vi "PhoenixLauncher.vi"() -> ()   [LabVIEW 2023]
uses:
  Vision_class/Old vision/Decode SSL and Refree Wrapper Package Folder/SSL Referee Game Status.ctl
  Vision_class/Old vision/Controls/SSL Field State.ctl
  Vision_class/Old vision/Controls/SSL Detection Frame.ctl
  Vision_class/Old vision/Controls/SSL Detection Robot.ctl
  <vilib>/Analysis/Matrix/Datatypes/RealMatrix.ctl
  Vision_class/Old vision/Controls/SSL Detection Ball.ctl
  Game_class/Game.lvclass
  Robot_class/robotDisplayFeedback.ctl
  <vilib>/Analysis/Matrix/NI_Matrix.lvlib
panel:
  out "String 2":string
  in  "Frame and Field Size out Ref":T1 {"Detection Frame Out"."robots_blue"."height" format="%+4.3f"; "Detection Frame Out"."robots_blue"."pixel_y" format="%+4.3f"; "Detection Frame Out"."robots_blue"."pixel_x" format="%+4.3f"; "Detection Frame Out"."robots_blue"."orientation" format="%+4.3f"; "Detection Frame Out"."robots_blue"."y" format="%+4.3f"; "Detection Frame Out"."robots_blue"."confidence" format="%4.3f"; "Detection Frame Out"."robots_blue"."x" format="%+4.3f"; "Detection Frame Out"."robots_yellow"."height" format="%+4.3f"; "Detection Frame Out"."robots_yellow"."pixel_y" format="%+4.3f"; "Detection Frame Out"."robots_yellow"."pixel_x" format="%+4.3f"; "Detection Frame Out"."robots_yellow"."orientation" format="%+4.3f"; "Detection Frame Out"."robots_yellow"."y" format="%+4.3f"; "Detection Frame Out"."robots_yellow"."confidence" format="%4.3f"; "Detection Frame Out"."robots_yellow"."x" format="%+4.3f"}
  in  "Field Size":T6
  in  "SSL Referee Game Status Ref":T7 {"Time" format="%<%.3X %x>T"; "Blue Timeout Remaining" format="%<%M:%S>t"; "Yellow Timeout Remaining" format="%<%M:%S>t"; "Time Left" format="%<%M:%S>t"}
  # "Score"
  # "Red Cards"
  # "Yellow Cards"
  # "Timeouts Left"
  # "Timeout Remaining"
  # "Goalie ID"
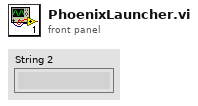
[diagram p1: front panel]
types:
  T1 = typedef "SSL Field State.ctl" = cluster{"Detection Frame Out":T2, "Field Size Out":cluster{"line_width":u32, "field_length":u32, "field_width":u32, "boundary_width":u32, "referee_width":u32, "goal_width":u32, "goal_depth":u32, "goal_wall_width":u32, "center_circle_radius":u32, "defense_radius":u32, "defense_stretch":u32, "free_kick_from_defense_dist":u32, "penalty_spot_from_field_line_dist":u32, "penalty_line_from_spot_dist":u32}, "Received Time Stamp":timestamp}
  T2 = typedef "SSL Detection Frame.ctl" = cluster{"frame_number":u32, "t_capture":dbl, "t_sent":dbl, "camera_id":u32, "robots_yellow":T3[], "robots_blue":T3[], "balls":T5[], "Valid":bool, "Time Stamp":timestamp, "New":bool, "Initialized":bool}
  T3 = typedef "SSL Detection Robot.ctl" = cluster{"x":sgl, "robot_id":u32, "confidence":sgl, "y":sgl, "orientation":sgl, "pixel_x":sgl, "pixel_y":sgl, "height":sgl, "Valid":bool, "Time Stamp":timestamp, "x_k|k":T4, "Pk|k":T4, "Previous Time Stamp":timestamp, "R":T4, "vx":dbl, "vy":dbl, "vang":dbl}
  T4 = typedef "NI_Matrix.lvlib/RealMatrix.ctl" = dbl[][]
  T5 = typedef "SSL Detection Ball.ctl" = cluster{"x":sgl, "area":u32, "confidence":sgl, "y":sgl, "z":sgl, "pixel_x":sgl, "pixel_y":sgl, "Valid":bool, "Time Stamp":timestamp, "x_k|k":T4, "Pk|k":T4, "Id":u32, "Previous Time Stamp":timestamp, "R":T4, " vx":sgl, "vy":dbl, "vz":dbl, " ax":sgl, "ay":dbl, "az":dbl}
  T6 = cluster{"line_width":u32, "field_length":u32, "field_width":u32, "boundary_width":u32, "referee_width":u32, "goal_width":u32, "goal_depth":u32, "goal_wall_width":u32, "center_circle_radius":u32, "defense_radius":u32, "defense_stretch":u32, "free_kick_from_defense_dist":u32, "penalty_spot_from_field_line_dist":u32, "penalty_line_from_spot_dist":u32}
  T7 = typedef "SSL Referee Game Status.ctl" = cluster{"Stage":string, "Command":string, "Time Left":dbl, "Yellow Team":string, "Blue Team":string, "Yellow Score":u32, "Blue Score":u32, "Yellow Red Cards":u32, "Blue Red Cards":u32, "Yellow Yellow Cards":u32, "Blue Yellow Cards":u32, "Yellow Timeouts Left":u32, "Blue Timeouts Left":u32, "Yellow Timeout Remaining":dbl, "Blue Timeout Remaining":dbl, "Yellow Goalie Id":u32, "Blue Goalie Id":u32, "Time":timestamp, "Point":cluster{"x":sgl, "y":sgl}}
  T8 = enum32{"Invalid", "Standard", "Closed", "Hidden", "Minimized", "Maximized"}
  T9 = typedef "robotDisplayFeedback.ctl" = cluster{"id":dbl, "encoder1":dbl, "encoder2":dbl, "kickCharge":bool, "ballInSensor":bool, "Battery (V)":dbl, "2D Picture":picture, "encoder3":dbl, "encoder4":dbl, "Valid":bool}
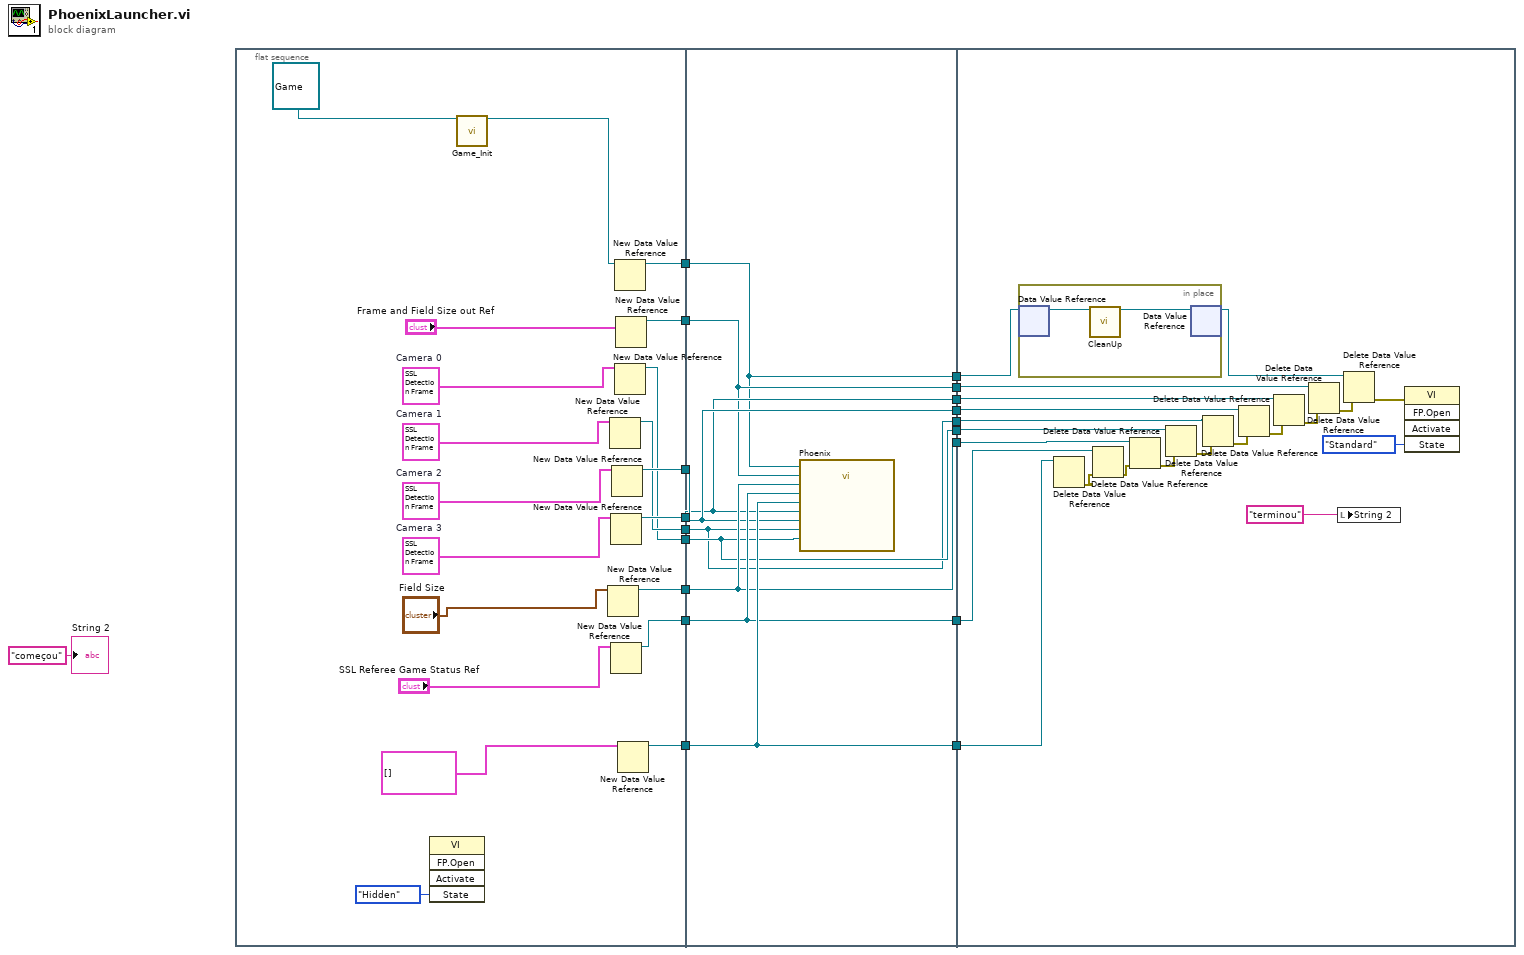
[diagram p0: block diagram]
diagram:
  n1 = flat-sequence {
    tunnel: [w29] -> w19
    tunnel: [w28] -> w18
    tunnel: [w27] -> w17
    tunnel: [w26] -> w16
    tunnel: [w25] -> w15
    tunnel: [w24] -> w14
    tunnel: [w23] -> w13
    tunnel: [w22] -> w12
    tunnel: [w21] -> w11
    tunnel: w19 -> [w40]
    tunnel: w18 -> [w41]
    tunnel: w17 -> [w46]
    tunnel: w16 -> [w47]
    tunnel: w15 -> [w48]
    tunnel: w14 -> [w42]
    tunnel: w13 -> [w43]
    tunnel: w12 -> [w44]
    tunnel: w11 -> [w45]
    tunnel: [w48] -> w10
    tunnel: [w47] -> w9
    tunnel: [w46] -> w8
    tunnel: [w45] -> w7
    tunnel: [w44] -> w6
    tunnel: [w43] -> w5
    tunnel: [w42] -> w4
    tunnel: [w41] -> w3
    tunnel: [w40] -> w2
    tunnel: w10 -> [w62]
    tunnel: w9 -> [w61]
    tunnel: w8 -> [w60]
    tunnel: w7 -> [w59]
    tunnel: w6 -> [w58]
    tunnel: w5 -> [w57]
    tunnel: w4 -> [w56]
    tunnel: w3 -> [w55]
    tunnel: w2 -> [w52]
    frame #0 {
      w33 = T2 {"frame_number"=0, "t_capture"=0.0, "t_sent"=0.0, "camera_id"=0, "robots_yellow"=[], "robots_blue"=[], "balls"=[], "Valid"=FALSE, "Time Stamp"=timestamp(0 s since 1904-01-01), "New"=FALSE, "Initialized"=FALSE}  # Camera 3
      w34 = T2 {"frame_number"=0, "t_capture"=0.0, "t_sent"=0.0, "camera_id"=0, "robots_yellow"=[], "robots_blue"=[], "balls"=[], "Valid"=FALSE, "Time Stamp"=timestamp(0 s since 1904-01-01), "New"=FALSE, "Initialized"=FALSE}  # Camera 2
      w35 = T2 {"frame_number"=0, "t_capture"=0.0, "t_sent"=0.0, "camera_id"=0, "robots_yellow"=[], "robots_blue"=[], "balls"=[], "Valid"=FALSE, "Time Stamp"=timestamp(0 s since 1904-01-01), "New"=FALSE, "Initialized"=FALSE}  # Camera 1
      w36 = T2 {"frame_number"=0, "t_capture"=0.0, "t_sent"=0.0, "camera_id"=0, "robots_yellow"=[], "robots_blue"=[], "balls"=[], "Valid"=FALSE, "Time Stamp"=timestamp(0 s since 1904-01-01), "New"=FALSE, "Initialized"=FALSE}  # Camera 0
      n2 = invoke class="VI" method="FP.Open"("State"=T8."Hidden") -> ()  [unwired: 4 in, 5 out]
      n3 = call "Game_Init.vi"("object in"=refnum<class "Game.lvclass"> refnum ("Game")) -> ("object out"=w38:refnum<class "Game.lvclass">)  [unwired: 17 in, 1 out]
      n4 = New Data Value Reference(data value="Field Size") -> (data value reference=w27:refnum<data-value>)  [unwired: 1 in, 1 out]
      n5 = New Data Value Reference(data value=w35) -> (data value reference=w22:refnum<data-value>)  [unwired: 1 in, 1 out]
      n6 = New Data Value Reference(data value=w33) -> (data value reference=w24:refnum<data-value>)  [unwired: 1 in, 1 out]
      n7 = New Data Value Reference(data value="SSL Referee Game Status Ref") -> (data value reference=w26:refnum<data-value>)  [unwired: 1 in, 1 out]
      n8 = New Data Value Reference(data value=w34) -> (data value reference=w23:refnum<data-value>)  [unwired: 1 in, 1 out]
      n9 = New Data Value Reference(data value=w38) -> (data value reference=w29:refnum<data-value>)  [unwired: 1 in, 1 out]
      n10 = New Data Value Reference(data value=w36) -> (data value reference=w21:refnum<data-value>)  [unwired: 1 in, 1 out]
      n11 = New Data Value Reference(data value="Frame and Field Size out Ref") -> (data value reference=w28:refnum<data-value>)  [unwired: 1 in, 1 out]
      n12 = New Data Value Reference(data value=T9[] [] ("displayFeedbackRobot 2")) -> (data value reference=w25:refnum<data-value>)  [unwired: 1 in, 1 out]
    }
    frame #1 {
      n13 = call "Phoenix.vi"("Game DVR"=w40, "Frame and Field Size out DVR"=w41, "Field Size DVR"=w46, "SSL Referee Game Status DVR"=w47, "Robot Display Feedback DVR"=w48, "Camera 0 DVR"=w45, "Camera 1 DVR"=w44, "Camera 2 DVR"=w43, "Camera 3 DVR"=w42) -> ()  [unwired: 11 in]
    }
    frame #2 {
      n14 = in-place {
        n15 = in-place-dvr #1(w52) -> (w71:refnum<class "Game.lvclass">)  [unwired: 1 out]
        n16 = call-dynamic "CleanUp.vi"("object in"=w71) -> ("object out"=w70:refnum<class "Game.lvclass">)  [unwired: 17 in, 1 out]
        n17 = in-place-dvr #1(w70) -> (w51:refnum<data-value>)  [unwired: 1 out]
      }
      n18 = Delete Data Value Reference(data value reference=w62) -> (error out=w65:errorcluster)  [unwired: 1 in, 1 out]
      n19 = Delete Data Value Reference(data value reference=w61, error in=w65) -> (error out=w66:errorcluster)  [unwired: 1 out]
      n20 = Delete Data Value Reference(data value reference=w60, error in=w66) -> (error out=w67:errorcluster)  [unwired: 1 out]
      n21 = Delete Data Value Reference(data value reference=w59, error in=w67) -> (error out=w68:errorcluster)  [unwired: 1 out]
      n22 = Delete Data Value Reference(data value reference=w58, error in=w68) -> (error out=w69:errorcluster)  [unwired: 1 out]
      n23 = Delete Data Value Reference(data value reference=w57, error in=w69) -> (error out=w64:errorcluster)  [unwired: 1 out]
      n24 = Delete Data Value Reference(data value reference=w56, error in=w64) -> (error out=w63:errorcluster)  [unwired: 1 out]
      n25 = Delete Data Value Reference(data value reference=w55, error in=w63) -> (error out=w54:errorcluster)  [unwired: 1 out]
      n26 = local write "String 2"("terminou" ("String")) -> ()
      n27 = Delete Data Value Reference(data value reference=w51, error in=w54) -> (error out=w53:errorcluster)  [unwired: 1 out]
      n28 = invoke class="VI" method="FP.Open"(error in=w53, "State"=T8."Standard") -> ()  [unwired: 3 in, 5 out]
    }
  }
  "String 2" <- "começou" ("String 2")
